vi "Receive Value Change Event.vi"(8 "error in (no error)":errorcluster, 10 "ValueChangeMsg":refnum<class "ValueChangeMsg.lvclass">, 11 "Entry Console View Definition In":refnum<class "Entry Console View Definition.lvclass">) -> (0 "error out":errorcluster, 3 "Entry Console View Definition Out":refnum<class "Entry Console View Definition.lvclass">)   [LabVIEW 2019, in "Entry Console View Definition.lvclass"]
doc: "<License>\nCopyright © 2017 Composed Systems, LLC | All rights reserved\nwww.composed.io\n\nAuthor: Ethan Stern <ethan.stern@composed.io>\n\nThis software is provided \"AS IS\" WITHOUT WARRANTIES, either express or implied, AND IS FOR EDUCATIONAL PURPOSES ONLY.\n</License>"
uses:
  <vilib>/gpm_packages/@cs/Car-wash/Source/Entry Console View Definition/Entry Console View Definition/Entry Console View Definition.lvclass
  <vilib>/gpm_packages/@cs/mva-viewable/Source/ActorEvents/IEventAggregator Messages/ValueChangeMsg/ValueChangeMsg.lvclass
  <vilib>/gpm_packages/@cs/mva-viewable/Source/ActorEvents/IEventAggregator Messages/ValueChangeMsg/ValueChangeMsg.lvclass/ValueChangeMsg.ctl
  <vilib>/gpm_packages/@cs/Car-wash/Source/Entry Console View Definition/Entry Console View Definition/Entry Console View Definition.lvclass/Entry Console View Definition.ctl
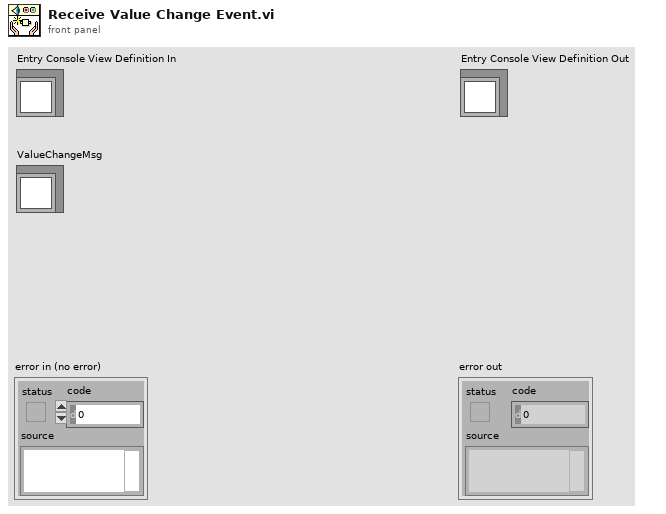
[diagram p1: front panel]
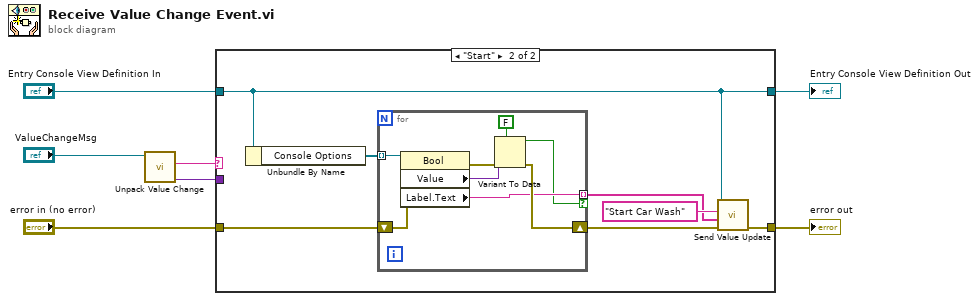
[diagram p0: block diagram]
diagram:
  n1 = call <vilib>:"Unpack Value Change.vi"("ValueChangeMsg"="ValueChangeMsg") -> ("New Value"=w1:variant, "Control Label"=w2:string)  [unwired: 6 in, 3 out]
  n2 = case shown="\"Start\"" w2 {
    tunnel: [w8 w16] -> w7
    tunnel: [w9 w14] -> w6
    tunnel: "error in (no error)" -> [w8 w13]
    tunnel: "Entry Console View Definition In" -> [w9 w14]
    tunnel: w1 -> [_ _]
    frame Default {
      # "Filter out events here"
    }
    frame "Start" {
      n3 = Unbundle By Name(w14) -> ("Console Options"=w11:refnum<vi>[])
      n4 = for {
        shift-right: [w20] -> w12
        shift-left: w13 -> [w21]
        tunnel: w11 -> [w24] mode=indexing
        tunnel: [w19] -> w10 mode=indexing if=w17
        n5 = property class="Bool"(reference=w24, error in=w21) -> (error out=w23:errorcluster, "Value"=w22:variant, "Label.Text"=w19:string)  [unwired: 1 out]
        n6 = Variant To Data(error in=w23, type=FALSE, Variant=w22) -> (data=w17:bool, error out=w20:errorcluster)
      }
      n7 = call-dynamic "Send Value Update.vi"("error in (no error)"=w12, "Value"=w10, "Datum Name"="Start Car Wash", "IViewable in"=w14) -> ("error out"=w16:errorcluster)  [unwired: 7 in]
    }
  }
  "error out" <- w7
  "Entry Console View Definition Out" <- w6
